vi "Gen_Fault_Dataset.vi"(9 "Number of Samples Per Class":i32=5000, 11 "Dataset Folder Path":path=path "D:/Ngene/Projects_SVN/DeepLTK/Examples/2_Waveform_Processing/24_Power_Transmission_Line_Fault_Classification/Dataset/Train") -> (3 "Dataset Folder Path":path=path "D:/Ngene/Projects_SVN/DeepLTK/Examples/2_Waveform_Processing/24_Power_Transmission_Line_Fault_Classification/Dataset/Train")   [LabVIEW 2020]
uses:
  <vilib>/Utility/file.llb/Write Delimited Spreadsheet (DBL).vi
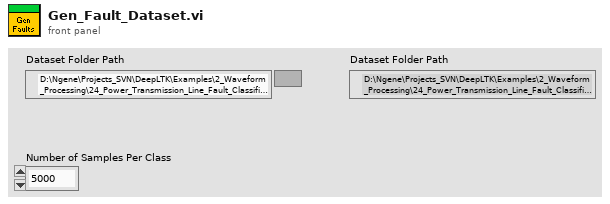
[diagram p1: front panel]
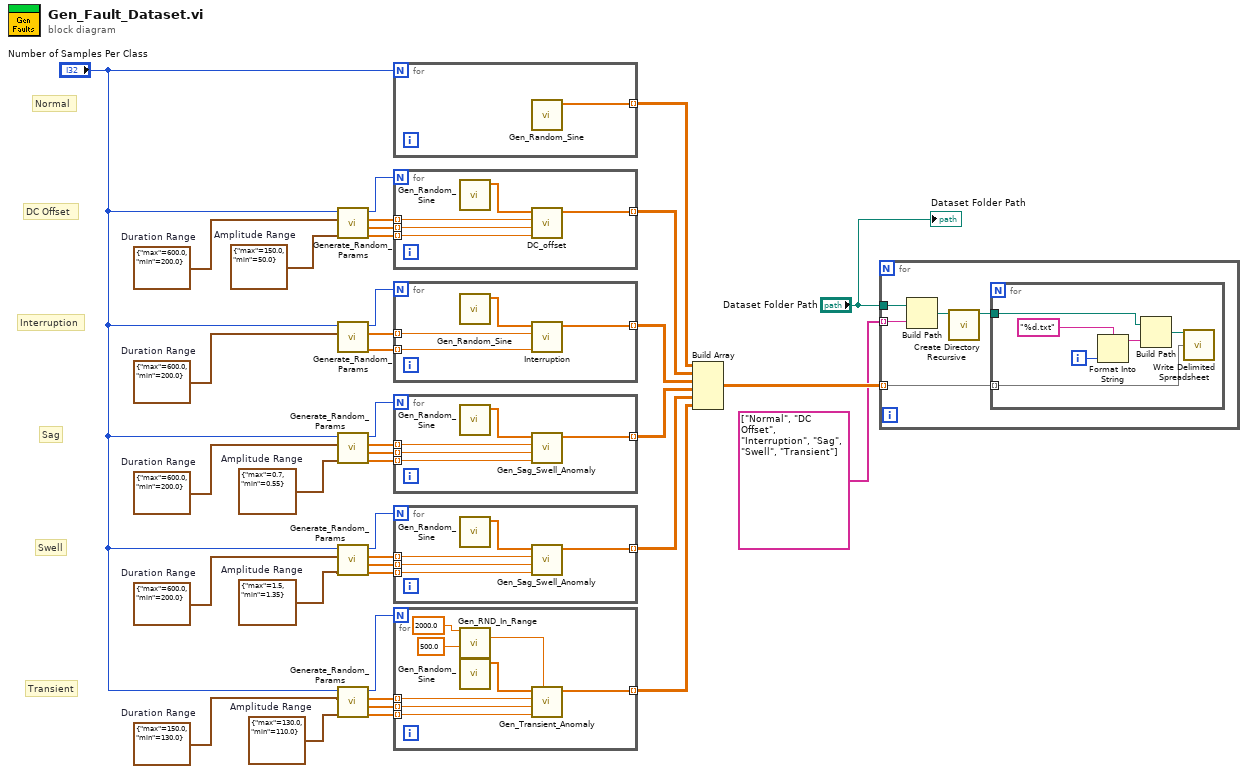
[diagram p0: block diagram]
diagram:
  w1 = cluster{"max":dbl, "min":dbl} {"max"=150.0, "min"=130.0}  # Duration Range
  w2 = cluster{"max":dbl, "min":dbl} {"max"=130.0, "min"=110.0}  # Amplitude Range
  w3 = cluster{"max":dbl, "min":dbl} {"max"=600.0, "min"=200.0}  # Duration Range
  w4 = cluster{"max":dbl, "min":dbl} {"max"=1.5, "min"=1.35}  # Amplitude Range
  w5 = cluster{"max":dbl, "min":dbl} {"max"=600.0, "min"=200.0}  # Duration Range
  w6 = cluster{"max":dbl, "min":dbl} {"max"=0.7, "min"=0.55}  # Amplitude Range
  w7 = cluster{"max":dbl, "min":dbl} {"max"=600.0, "min"=200.0}  # Duration Range
  w8 = cluster{"max":dbl, "min":dbl} {"max"=600.0, "min"=200.0}  # Duration Range
  w9 = cluster{"max":dbl, "min":dbl} {"max"=150.0, "min"=50.0}  # Amplitude Range
  # "Normal"
  # "Swell"
  # "DC Offset"
  # "Interruption"
  # "Sag"
  # "Transient"
  n1 = call "Generate_Random_Params.vi"("Amplitude Range"=w9, "Duration Range"=w8, "Samples"="Number of Samples Per Class") -> ("Duration"=w19:dbl[], "Amplitude"=w20:dbl[], "Position"=w21:dbl[], "Samples"=w18:i32)  [unwired: 5 in]
  n2 = call "Generate_Random_Params.vi"("Duration Range"=w7, "Samples"="Number of Samples Per Class") -> ("Duration"=w24:dbl[], "Position"=w25:dbl[], "Samples"=w23:i32)  [unwired: 6 in, 1 out]
  n3 = call "Generate_Random_Params.vi"("Amplitude Range"=w6, "Duration Range"=w5, "Samples"="Number of Samples Per Class") -> ("Duration"=w29:dbl[], "Amplitude"=w28:dbl[], "Position"=w27:dbl[], "Samples"=w30:i32)  [unwired: 5 in]
  n4 = call "Generate_Random_Params.vi"("Amplitude Range"=w4, "Duration Range"=w3, "Samples"="Number of Samples Per Class") -> ("Duration"=w32:dbl[], "Amplitude"=w33:dbl[], "Position"=w34:dbl[], "Samples"=w31:i32)  [unwired: 5 in]
  n5 = call "Generate_Random_Params.vi"("Amplitude Range"=w2, "Duration Range"=w1, "Samples"="Number of Samples Per Class") -> ("Duration"=w11:dbl[], "Amplitude"=w10:dbl[], "Position"=w14:dbl[], "Samples"=w15:i32)  [unwired: 5 in]
  n6 = for {
    N: "Number of Samples Per Class" -> [_]
    tunnel: [w39] -> w16 mode=indexing
    n7 = call "Gen_Random_Sine.vi"() -> ("data"=w39:dbl[])  [unwired: 11 in]
  }
  n8 = for {
    N: w18 -> [_]
    tunnel: [w44] -> w17 mode=indexing
    tunnel: w21 -> [w43] mode=indexing
    tunnel: w20 -> [w42] mode=indexing
    tunnel: w19 -> [w41] mode=indexing
    n9 = call "Gen_Random_Sine.vi"() -> ("data"=w40:dbl[])  [unwired: 11 in]
    n10 = call "DC_offset.vi"("Duration"=w41, "Ampltude"=w42, "Position"=w43, "Sine"=w40) -> ("Sine+Anomaly"=w44:sgl[])  [unwired: 7 in]
  }
  n11 = for {
    N: w23 -> [_]
    tunnel: [w48] -> w22 mode=indexing
    tunnel: w25 -> [w47] mode=indexing
    tunnel: w24 -> [w46] mode=indexing
    n12 = call "Gen_Random_Sine.vi"() -> ("data"=w45:dbl[])  [unwired: 11 in]
    n13 = call "Interruption.vi"("Duration"=w46, "Position"=w47, "Sine"=w45) -> ("Sine+Anomaly"=w48:sgl[])  [unwired: 8 in]
  }
  n14 = for {
    N: w30 -> [_]
    tunnel: [w53] -> w26 mode=indexing
    tunnel: w27 -> [w52] mode=indexing
    tunnel: w28 -> [w51] mode=indexing
    tunnel: w29 -> [w50] mode=indexing
    n15 = call "Gen_Random_Sine.vi"() -> ("data"=w49:dbl[])  [unwired: 11 in]
    n16 = call "Gen_Sag_Swell_Anomaly.vi"("Duration"=w50, "Amplitude"=w51, "Position"=w52, "Sine"=w49) -> ("Sine+Anomaly"=w53:sgl[])  [unwired: 7 in]
  }
  n17 = for {
    N: w31 -> [_]
    tunnel: [w58] -> w38 mode=indexing
    tunnel: w34 -> [w57] mode=indexing
    tunnel: w33 -> [w56] mode=indexing
    tunnel: w32 -> [w55] mode=indexing
    n18 = call "Gen_Random_Sine.vi"() -> ("data"=w54:dbl[])  [unwired: 11 in]
    n19 = call "Gen_Sag_Swell_Anomaly.vi"("Duration"=w55, "Amplitude"=w56, "Position"=w57, "Sine"=w54) -> ("Sine+Anomaly"=w58:sgl[])  [unwired: 7 in]
  }
  n20 = for {
    N: w15 -> [_]
    tunnel: [w66] -> w12 mode=indexing
    tunnel: w14 -> [w65] mode=indexing
    tunnel: w11 -> [w63] mode=indexing
    tunnel: w10 -> [w59] mode=indexing
    n21 = call "Gen_RND_In_Range.vi"("Upper Bound"=2000.0 ("frequency"), "Lower Bound"=500.0 ("Variation%")) -> ("RND_In_Range"=w60:dbl)  [unwired: 13 in]
    n22 = call "Gen_Random_Sine.vi"() -> ("data"=w64:dbl[])  [unwired: 11 in]
    n23 = call "Gen_Transient_Anomaly.vi"("Frequency"=w60, "Tau"=w63, "Amplitude"=w59, "Position"=w65, "Sine"=w64) -> ("Sine+Anomaly"=w66:sgl[])  [unwired: 6 in]
  }
  n24 = Build Array(w16, w17, w22, w26, w38, w12) -> (w37:dbl[][][])
  n25 = for {
    tunnel: w37 -> [w71] mode=indexing
    tunnel: "Dataset Folder Path" -> [w70]
    tunnel: string[] ["Normal", "DC Offset", "Interruption", "Sag", "Swell", "Transient"] -> [w68] mode=indexing
    n26 = Build Path(base path=w70, name or relative path=w68) -> (appended path=w69:path)
    n27 = call <vilib>:"Create Directory Recursive.vi"("directory"=w69) -> ("directory copy"=w67:path)  [unwired: 4 in, 2 out]
    n28 = for {
      tunnel: w71 -> [w76] mode=indexing
      tunnel: w67 -> [w77]
      i -> [w73]
      n29 = Format Into String(format string="%d.txt", w73) -> (resulting string=w72:string)  [unwired: 2 in, 1 out]
      n30 = Build Path(base path=w77, name or relative path=w72) -> (appended path=w75:path)
      n31 = call-poly <vilib>:"Write Delimited Spreadsheet.vi"("file path (dialog if empty)"=w75, "1D data"=w76) -> ()  [unwired: 12 in, 2 out]
    }
  }
  "Dataset Folder Path" <- "Dataset Folder Path"
